vi "Config_K2400.vi"(8 "error in":errorcluster) -> (0 "error out 2":errorcluster)   [LabVIEW 2020]
uses:
  <instrlib>/Keithley 24XX/Keithley 24XX.lvlib
panel:
  in  "Reset (True)":bool=TRUE
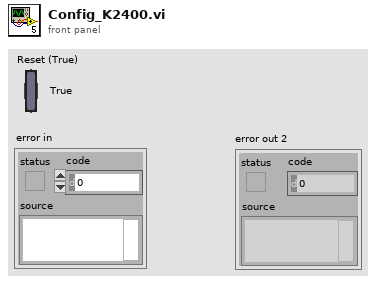
[diagram p1: front panel]
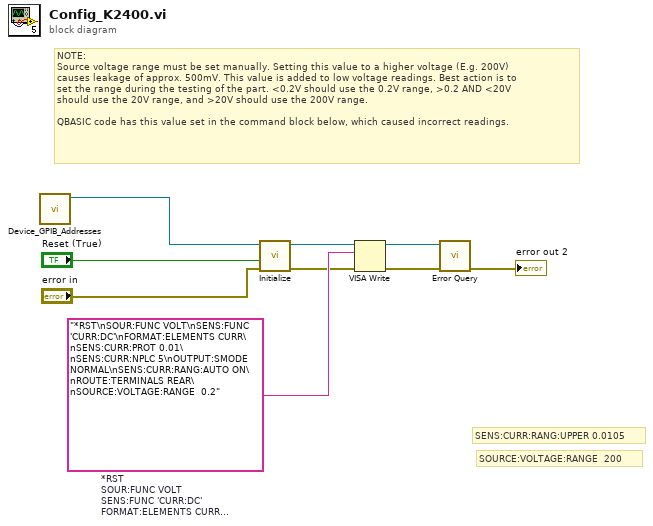
[diagram p0: block diagram]
diagram:
  w7 = "*RST\nSOUR:FUNC VOLT\nSENS:FUNC 'CURR:DC'\nFORMAT:ELEMENTS CURR\nSENS:CURR:PROT 0.01\nSENS:CURR:NPLC 5\nOUTPUT:SMODE NORMAL\nSENS:CURR:RANG:AUTO ON\nROUTE:TERMINALS REAR\nSOURCE:VOLTAGE:RANGE  0.2"  # *RST SOUR:FUNC VOLT SENS:FUNC 'CURR:DC' FORMAT:ELEMENTS CURR SENS:CURR:PROT 0.01 SENS:CURR:NPLC 5 OUTPUT:SMODE NORMAL SENS:CURR:RANG:AUTO ON ROUTE:TERMINALS REAR SOURCE:VOLTAGE:RANGE  0.2
  # "SOURCE:VOLTAGE:RANGE  200"
  # "SENS:CURR:RANG:UPPER 0.0105"
  # "NOTE:\nSource voltage range must be set manually. Setting this value to a higher voltage (E.g. 200V)\ncauses leakage of approx. 500mV. This value is added to low voltage readings. Best action is to\nset the range during the testing of the part. <0.2V should use the 0.2V range, >0.2 AND <20V\nshould use the 20V range, and >20V should use the 200V range.\n\nQBASIC code has this value set in the command block below, which caused incorrect readings."
  n1 = call "Device_GPIB_Addresses.vi"() -> ("Keithley 2400 Address"=w1:refnum<visa-resource-name>)  [unwired: 9 in, 2 out]
  n2 = call <instrlib>:"Initialize.vi"("error in (no error)"="error in", "Reset (True)"="Reset (True)", "VISA resource name"=w1) -> ("error out"=w2:errorcluster, "VISA resource name out"=w3:refnum<visa-resource-name>)  [unwired: 7 in]
  n3 = VISA Write(VISA resource name=w3, write buffer=w7, error in (no error)=w2) -> (VISA resource name out=w5:refnum<visa-resource-name>, error out=w4:errorcluster)  [unwired: 1 out]
  n4 = call <instrlib>:"Error Query.vi"("error in (no error)"=w4, "VISA resource name"=w5) -> ("error out"=→"error out 2":errorcluster)  [unwired: 6 in, 3 out]
